vi "Write shutdown action config.vi"(8 "error in (no error)":errorcluster, 10 "shutdown action config":refnum<class "action configuration.lvclass">, 11 "Simple Sequencer TBM configuration in":refnum<class "Simple Sequencer TBM configuration.lvclass">) -> (0 "error out":errorcluster, 3 "Simple Sequencer TBM configuration out":refnum<class "Simple Sequencer TBM configuration.lvclass">)   [LabVIEW 2014, in "Simple Sequencer TBM configuration.lvclass"]
uses:
  Simple Sequencer TBM configuration.lvclass
  sequencer parent classes/action configuration parent/action configuration.lvclass
  Simple Sequencer TBM configuration.lvclass/Simple Sequencer TBM configuration.ctl
  <vilib>/NI/Configuration Framework/serializable configuration/NISE_CEF_serializable configuration.lvclass
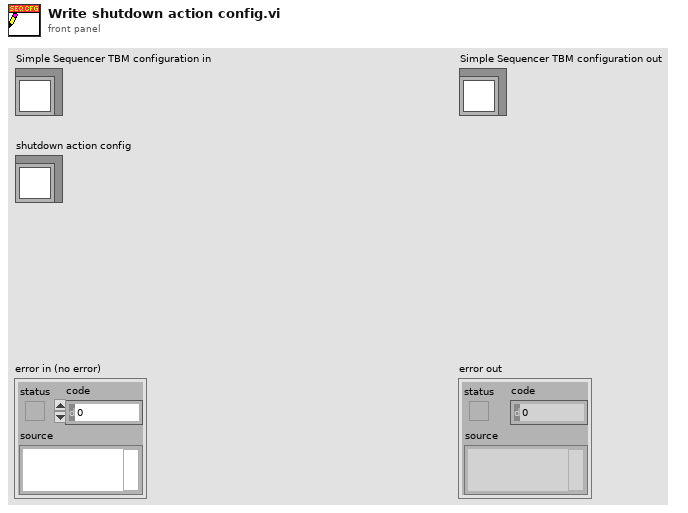
[diagram p1: front panel]
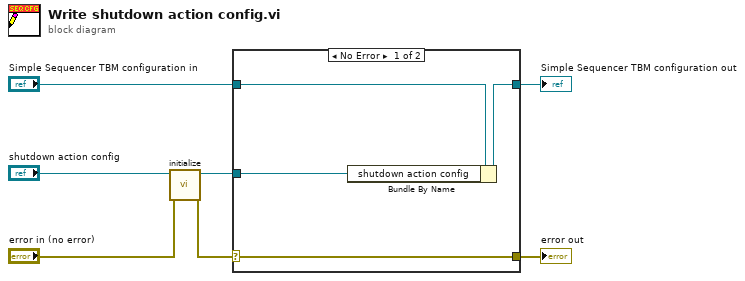
[diagram p0: block diagram]
diagram:
  n1 = call <vilib>:"initialize.vi"("error in"="error in (no error)", "configuration in"="shutdown action config") -> ("error out"=w1:errorcluster, "configuration out"=w3:refnum<class "action configuration.lvclass">)  [unwired: 7 in, 1 out]
  n2 = case shown="No Error" w1 {
    selector: w1 -> [w11 w12]
    tunnel: [w11 w12] -> w7
    tunnel: [w9 w13] -> w5
    tunnel: "Simple Sequencer TBM configuration in" -> [w10 w13]
    tunnel: w3 -> [w8 _]
    frame No Error {
      n3 = Bundle By Name(cluster=w10, "shutdown action config"=w8) -> (w9:refnum<class "Simple Sequencer TBM configuration.lvclass">)
    }
    frame Error {
    }
  }
  "error out" <- w7
  "Simple Sequencer TBM configuration out" <- w5
